vi "Destroy.vi"(8 "Error In":errorcluster, 11 "Graph In":refnum<class "Graph.lvclass">) -> (0 "Error Out":errorcluster)   [LabVIEW 2019, in "Graph.lvclass"]
uses:
  Graph.lvclass
  Display Element/Display Element.lvclass
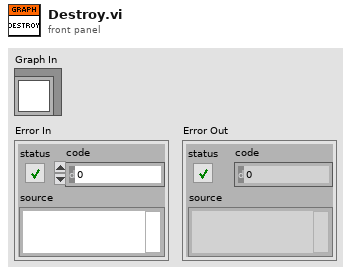
[diagram p1: front panel]
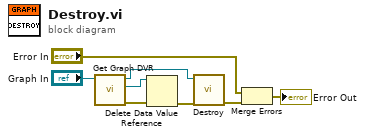
[diagram p0: block diagram]
diagram:
  n1 = call "Get Graph DVR.vi"("Graph In"="Graph In") -> ("Error Out"=w4:errorcluster, "DVR"=w8:refnum<data-value>, "Graph Out"=w6:refnum<class "Graph.lvclass">)  [unwired: 8 in]
  n2 = Delete Data Value Reference(data value reference=w8, error in=w4) -> (error out=w5:errorcluster)  [unwired: 1 out]
  n3 = call-parent "Destroy.vi"("Error In"=w5, "Display Element In"=w6) -> ("Error Out"=w2:errorcluster)  [unwired: 9 in]
  n4 = Merge Errors("Error In", w2) -> (→"Error Out":errorcluster)
